vi "TCP Reception Loop.vi"(7 "Array 2":u16[](array[numeric]), 10 "address":string, 11 "output cluster":T2) -> ()   [LabVIEW 2016]
uses:
  <vilib>/vision/Image Controls.llb/IMAQ Image.ctl
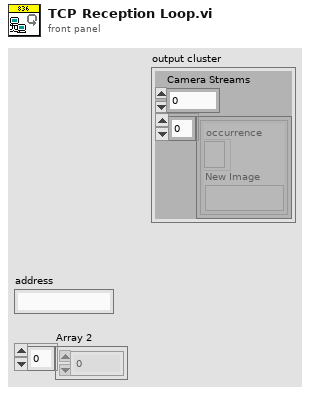
[diagram p1: front panel]
types:
  T1 = typedef "IMAQ Image.ctl" = refnum<image>
  T2 = cluster{"Camera Streams":i32, cluster{"occurrence":refnum<k4>, "New Image":T1}[]}
  T3 = cluster{"occurrence":refnum<k4>, "New Image":T1}[]
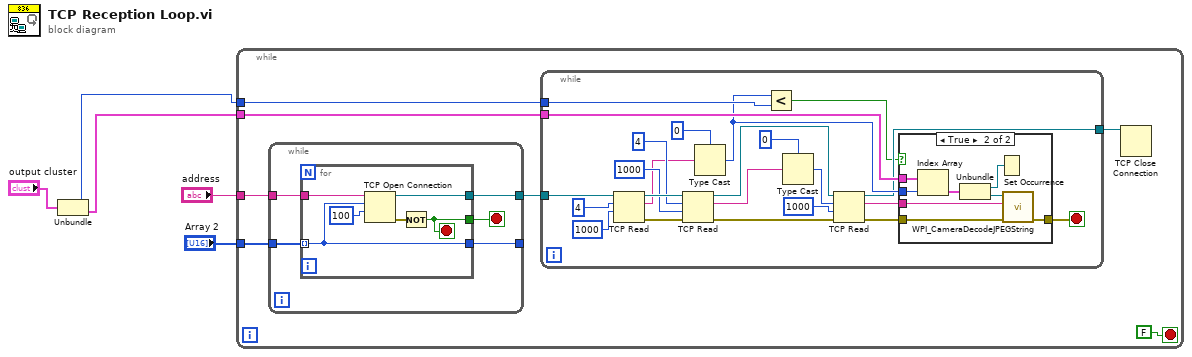
[diagram p0: block diagram]
diagram:
  n1 = Unbundle("output cluster") -> ("Camera Streams"=w1:i32, w2:T3)
  n2 = while {
    tunnel: "Array 2" -> [w12]
    tunnel: w2 -> [w8]
    tunnel: w1 -> [w7]
    tunnel: "address" -> [w6]
    stop <- FALSE stop-if-true
    n3 = while {
      tunnel: w12 -> [w49]
      tunnel: [w47] -> w10
      tunnel: [w46] -> _
      tunnel: w6 -> [w45]
      stop <- w48 stop-if-true
      n4 = for {
        tunnel: w49 -> [w51] mode=indexing
        tunnel: [w53] -> w48
        tunnel: [w52] -> w47
        tunnel: [w51] -> w46
        tunnel: w45 -> [w50]
        stop <- w53 stop-if-true
        n5 = TCP Open Connection(address=w50, remote port or service name=w51, timeout ms (60000)=100) -> (connection ID=w52:refnum<k5>, error out=w54:errorcluster)  [unwired: 2 in]
        n6 = Not(x=w54) -> (.not. x?=w53:bool)
      }
    }
    n7 = while {
      tunnel: w10 -> [w35]
      tunnel: [w14] -> w9
      tunnel: w8 -> [w17]
      tunnel: w7 -> [w16]
      stop <- w19 stop-if-true
      n8 = TCP Read(connection ID=w35, bytes to read=4, 9:1000 ("timeout ms (25000)")) -> (connection ID out=w31:refnum<k5>, data out=w23:string, error out=w32:errorcluster)  [unwired: 2 in]
      n9 = TCP Read(connection ID=w31, bytes to read=4, error in (no error)=w32, 9:1000 ("timeout ms (25000)")) -> (connection ID out=w18:refnum<k5>, data out=w29:string, error out=w24:errorcluster)  [unwired: 1 in]
      n10 = Type Cast(type=0 ("bytes to read"), x=w23) -> (*(type *) &x=w15:i32)
      n11 = Less?(x=w15, y=w16) -> (x < y?=w13:bool)
      n12 = Type Cast(type=0 ("bytes to read"), x=w29) -> (*(type *) &x=w27:i32)
      n13 = TCP Read(connection ID=w18, bytes to read=w27, error in (no error)=w24, 9:1000 ("timeout ms (25000)")) -> (connection ID out=w14:refnum<k5>, data out=w21:string, error out=w20:errorcluster)  [unwired: 1 in]
      n14 = case shown="True" w13 {
        tunnel: w21 -> [_ w44]
        tunnel: w20 -> [w36 w43]
        tunnel: [w36 w42] -> w19
        tunnel: w17 -> [_ w41]
        tunnel: w15 -> [_ w37]
        frame False {
        }
        frame True {
          n15 = Index Array(array=w41, index=w37) -> (element=w40:cluster{"occurrence":refnum<k4>, "New Image":T1})
          n16 = Unbundle(w40) -> ("occurrence"=w38:refnum<k4>, "New Image"=w39:T1)
          n17 = Set Occurrence(w38) -> ()
          n18 = call <vilib>:"WPI_CameraDecodeJPEGString.vi"("error in"=w43, "Compressed Image"=w44, "Image In"=w39) -> ("error out"=w42:errorcluster)  [unwired: 4 out]
        }
      }
    }
    n19 = TCP Close Connection(connection ID=w9) -> ()  [unwired: 2 in, 2 out]
  }
